vi "ExposeToCSComNPMessage.vi"(11 "Message":T1 {"Message Type" items=["Error"=1, "Warning"=2, "Create"=4, "Destroy"=8, "Invoke"=16, "Get"=32, "Set"=64, "Response"=128]}) -> (3 ".NET Refnum out":refnum<k24>)   [LabVIEW 2017]
uses:
  C:/Code/CMCryoSysCode/Expose/COM/CSCom/CSCom/bin/Release/CSCom.dll
  COM/CSCom/CSCom/bin/Release/CSCom.dll
  ExposeMessage.ctl
  Events/ExposeMessageType.ctl
  Mapper/ExposeObjectMapNamepathData.ctl
  Mapper/ExposeMapperDataTypeEnum.ctl
  Mapper/ExposeObjectMapContainerTypeEnum.ctl
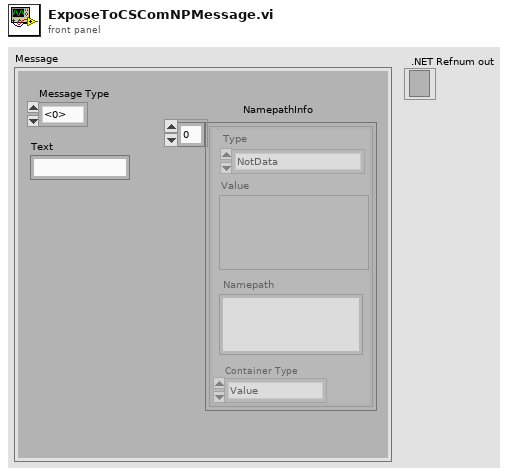
[diagram p1: front panel]
types:
  T1 = typedef "ExposeMessage.ctl" = cluster{"Message Type":T2, "Text":string, "NamepathInfo":T3[]}
  T2 = typedef "ExposeMessageType.ctl" = i32
  T3 = typedef "ExposeObjectMapNamepathData.ctl" = cluster{"Type":T4, "Value":variant, "Namepath":string, "Container Type":T5}
  T4 = typedef "ExposeMapperDataTypeEnum.ctl" = enum16{"NotData", "int8", "byte", "int16", "uint16", "int32", "uint32", "int64", "uint64", "Single", "Double", "String", "Boolean", "Container"}
  T5 = typedef "ExposeObjectMapContainerTypeEnum.ctl" = enum16{"Value", "Array", "Waveform", "NetContainer"}
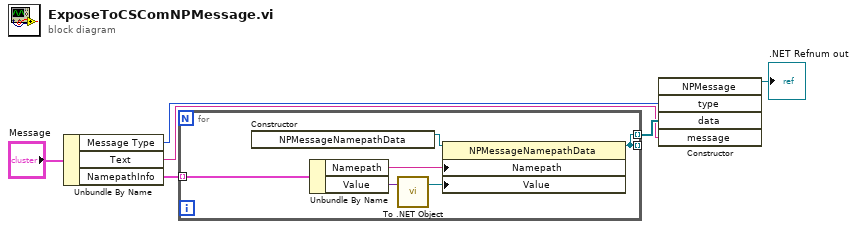
[diagram p0: block diagram]
diagram:
  n1 = Unbundle By Name("Message") -> ("Message Type"=w2:T2, "Text"=w3:string, "NamepathInfo"=w4:T3[])
  n2 = for {
    tunnel: w4 -> [w12] mode=indexing
    tunnel: [w7] -> _ mode=indexing
    tunnel: [w7] -> w5 mode=indexing
    n3 = constructor class="NPMessageNamepathData"() -> (reference out=w8:refnum<k24>)  [unwired: 3 in, 2 out]
    n4 = Unbundle By Name(w12) -> ("Namepath"=w9:string, "Value"=w11:variant)
    n5 = call <vilib>:"To .NET Object.vi"("anything"=w11) -> (".NET object"=w10:refnum<k24>)  [unwired: 1 in, 1 out]
    n6 = property class="NPMessageNamepathData"(reference=w8, "Namepath"=w9, "Value"=w10) -> (reference out=w7:refnum<k24>)  [unwired: 1 in, 1 out]
  }
  n7 = constructor class="NPMessage"("type"=w2, "data"=w5, "message"=w3) -> (reference out=→".NET Refnum out":refnum<k24>)  [unwired: 3 in, 5 out]
